vi "Add Major Frame.vi"(8 "error in":errorcluster, 9 "minorFrames":string[](array[string]), 10 "name":string, 11 "channel in":refnum<k24>) -> (0 "error out":errorcluster, 2 "new major frame":refnum<k24>, 3 "channel out":refnum<k24>)   [LabVIEW 2020, in "Ballard_1553_Parameter_ni.lvlib"]
uses:
  Ballard_1553_Parameter_ni.lvlib
  C:/Users/Administrator/Desktop/GIT/Ballard-Arinc-429-XML-Generator/Source/Assemblies/Aim_1553_Parameter_ni/bin/Debug/AIM_1553_Parameter_ni.dll
  Assemblies/Aim_1553_Parameter_ni/bin/Debug/AIM_1553_Parameter_ni.dll
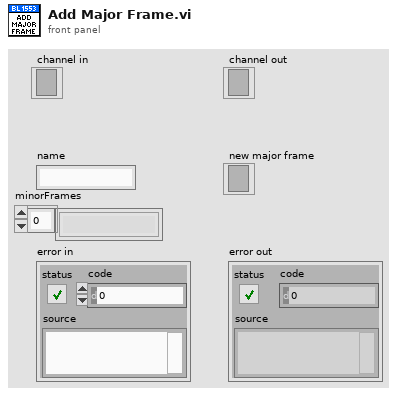
[diagram p1: front panel]
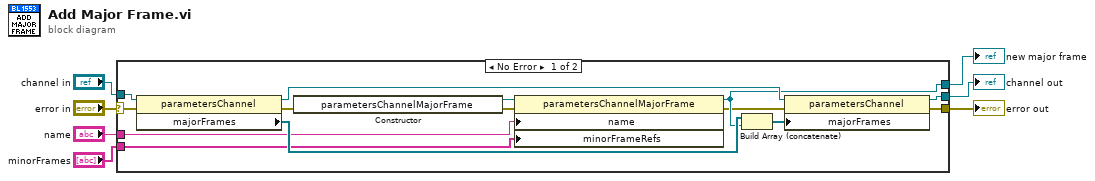
[diagram p0: block diagram]
diagram:
  n1 = case shown="No Error" "error in" {
    selector: "error in" -> [w20 w22]
    tunnel: [w17 w23] -> w7
    tunnel: [w16 w22] -> w6
    tunnel: "channel in" -> [w21 w23]
    tunnel: [w10 _] -> w2
    tunnel: "name" -> [w11 _]
    tunnel: "minorFrames" -> [w8 _]
    frame No Error {
      n2 = property class="parametersChannel"(reference=w21, error in=w20) -> (reference out=w18:refnum<k24>, error out=w13:errorcluster, "majorFrames"=w19:refnum<k24>[])
      n3 = constructor class="parametersChannelMajorFrame"(error in=w13) -> (reference out=w12:refnum<k24>, error out=w14:errorcluster)  [unwired: 2 in, 1 out]
      n4 = property class="parametersChannelMajorFrame"(reference=w12, error in=w14, "name"=w11, "minorFrameRefs"=w8) -> (reference out=w10:refnum<k24>, error out=w9:errorcluster)
      n5 = Build Array (concatenate)(w19, w10) -> (w15:refnum<k24>[])
      n6 = property class="parametersChannel"(reference=w18, error in=w9, "majorFrames"=w15) -> (reference out=w17:refnum<k24>, error out=w16:errorcluster)
    }
    frame Error {
    }
  }
  "channel out" <- w7
  "error out" <- w6
  "new major frame" <- w2
